vi "DMA Read-Windows Host.vi"() -> ()   [LabVIEW 2012]
uses:
  <vilib>/rvi/interface/RandomDataEmulation/nirviRandomDataOpen.vi
  <vilib>/rvi/interface/RandomDataEmulation/nirviRandomDataDMAMethods.vi
  <vilib>/rvi/interface/RandomDataEmulation/niFpgaReadControlTemplate.vi
  <vilib>/rvi/interface/RandomDataEmulation/niFpgaWriteControlTemplate.vi
  <vilib>/rvi/interface/RandomDataEmulation/nirviRandomDataClose.vi
  <vilib>/rvi/interface/nirviOpenFPGA/nirviOpenFPGA.xnode
  DMA Write-FPGA.vi
  <vilib>/rvi/interface/nirviMethod/nirviMethod.xnode
  <vilib>/rvi/interface/nirviReadWriteControl/nirviReadWriteControl.xnode
  <vilib>/rvi/interface/nirviCloseFPGA/nirviCloseFPGA.xnode
panel:
  out "Flushed Data":i16[](array[numeric])
  out "Overflow Count":u32
  out "Data":i16[](graph)
  out "error out":errorcluster
  in  "stop":bool
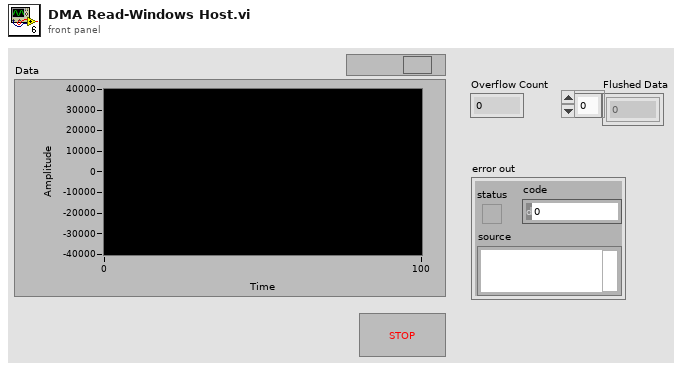
[diagram p1: front panel]
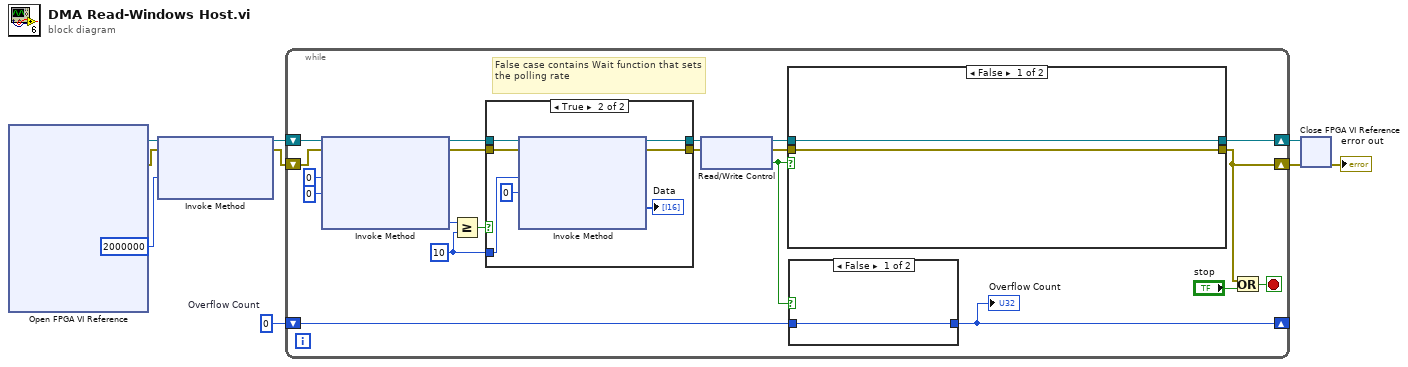
[diagram p0: block diagram]
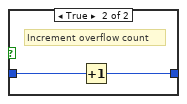
[diagram p2: hidden frame]
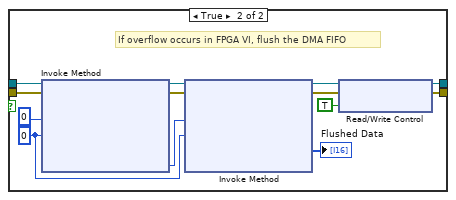
[diagram p3: hidden frame]
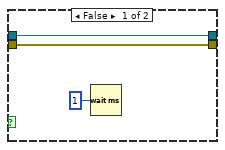
[diagram p4: hidden frame]
diagram:
  w5 = u32 0  # Overflow Count
  n1 = xnode "Open FPGA VI Reference"() -> ("FPGA VI Reference Out"=w2:refnum<k20>, "error out"=w1:errorcluster)  [unwired: 2 in]
  n2 = xnode "Invoke Method"("FPGA VI Reference In"=w2, "error in"=w1, "Requested Depth"=u32 2000000 ("Depth")) -> ("FPGA VI Reference Out"=w3:refnum<k20>, "error out"=w4:errorcluster)  [unwired: 1 out]
  n3 = while {
    shift-right: [w10] -> w9
    shift-left: w3 -> [w29]
    shift-right: [w14] -> w8
    shift-left: w4 -> [w28]
    shift-right: [w15] -> _
    shift-left: w5 -> [w16]
    stop <- w12 stop-if-true
    w25 = u32 10 ("y")
    # "False case contains Wait function that sets the polling rate"
    n4 = xnode "Invoke Method"("FPGA VI Reference In"=w29, "error in"=w28, "Number of Elements"=u32 0, "Timeout (ms)"=0) -> ("FPGA VI Reference Out"=w24:refnum<k20>, "error out"=w23:errorcluster, "Elements Remaining"=w27:u32)  [unwired: 1 out]
    n5 = Greater Or Equal?(x=w27, y=w25) -> (x >= y?=w26:bool)
    n6 = case shown="True" w26 {
      tunnel: w25 -> [_ w57]
      tunnel: w24 -> [w50 w55]
      tunnel: w23 -> [w49 w54]
      tunnel: [w50 w53] -> w11
      tunnel: [w49 w52] -> w20
      frame False {
        n7 = Wait (ms)(milliseconds to wait=u32 1) -> ()  [unwired: 1 out]
      }
      frame True {
        n8 = xnode "Invoke Method"("FPGA VI Reference In"=w55, "error in"=w54, "Number of Elements"=w57, "Timeout (ms)"=0) -> ("FPGA VI Reference Out"=w53:refnum<k20>, "error out"=w52:errorcluster, "Data"=→"Data":i16[])  [unwired: 1 out]
      }
    }
    n9 = xnode "Read/Write Control"("FPGA VI Reference In"=w11, "error in"=w20) -> ("FPGA VI Reference Out"=w19:refnum<k20>, "error out"=w18:errorcluster, "Overflow?"=w17:bool)
    n10 = case shown="False" w17 {
      tunnel: w19 -> [w34 w47]
      tunnel: w18 -> [w33 w46]
      tunnel: [w34 w40] -> w10
      tunnel: [w33 w39] -> w14
      frame False {
      }
      frame True {
        w36 = 0 ("Timeout (ms)")
        # "If overflow occurs in FPGA VI, flush the DMA FIFO"
        n11 = xnode "Invoke Method"("FPGA VI Reference In"=w47, "error in"=w46, "Number of Elements"=u32 0, "Timeout (ms)"=w36) -> ("FPGA VI Reference Out"=w45:refnum<k20>, "error out"=w44:errorcluster, "Elements Remaining"=w37:u32)  [unwired: 1 out]
        n12 = xnode "Invoke Method"("FPGA VI Reference In"=w45, "error in"=w44, "Number of Elements"=w37, "Timeout (ms)"=w36) -> ("FPGA VI Reference Out"=w42:refnum<k20>, "error out"=w41:errorcluster, "Data"=→"Flushed Data":i16[])  [unwired: 1 out]
        n13 = xnode "Read/Write Control"("FPGA VI Reference In"=w42, "error in"=w41, "DMA Cleared?"=TRUE ("Reset")) -> ("FPGA VI Reference Out"=w40:refnum<k20>, "error out"=w39:errorcluster)
      }
    }
    n14 = case shown="False" w17 {
      tunnel: w16 -> [w30 w32]
      tunnel: [w30 w31] -> w15
      frame False {
      }
      frame True {
        # "Increment overflow count"
        n15 = Increment(x=w32) -> (x+1=w31:u32)
      }
    }
    "Overflow Count" <- w15
    n16 = Or(x=w14, y="stop") -> (x .or. y?=w12:bool)
  }
  n17 = xnode "Close FPGA VI Reference"("FPGA VI Reference In"=w9, "error in"=w8) -> ("error out"=→"error out":errorcluster)
